vi "RCL.vi"(8 "error in (no error)":errorcluster, 10 "Memory":T1, 11 "refnum in":T2) -> (3 "refnum out":T2, 4 "question out":string)   [LabVIEW 2021, in "Korad KA3305P.lvlib"]
uses:
  Korad KA3305P.lvlib
  Reference.ctl
  MemoryNo.ctl
panel:
  out "error out":errorcluster
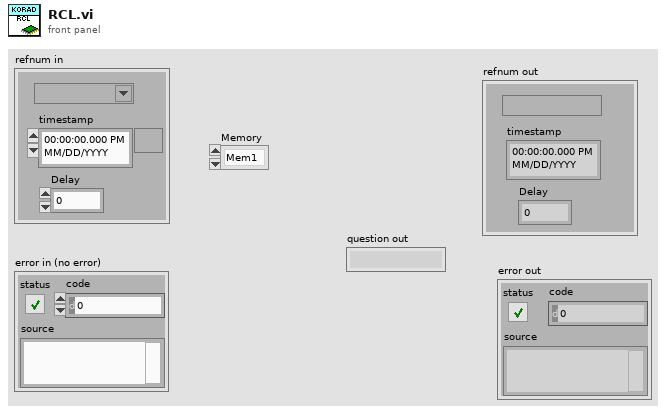
[diagram p1: front panel]
types:
  T1 = typedef "Korad KA3305P.lvlib/MemoryNo.ctl" = enum16{"Mem1", "Mem2", "Mem3", "Mem4", "Mem5"}
  T2 = typedef "Korad KA3305P.lvlib/Reference.ctl" = cluster{"refnum":refnum<visa-resource-name>, "timestamp":timestamp, "Delay":dbl}
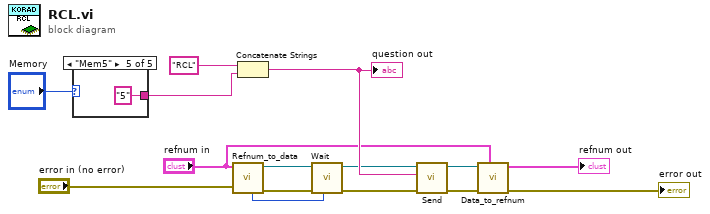
[diagram p0: block diagram]
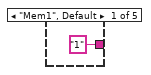
[diagram p2: hidden frame]
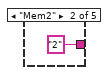
[diagram p3: hidden frame]
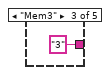
[diagram p4: hidden frame]
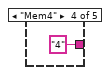
[diagram p5: hidden frame]
diagram:
  n1 = case shown="\"Mem5\"" "Memory" {
    tunnel: ["1" ("string") "2" ("string") "3" ("string") "4" ("string") "5" ("string")] -> w1
    frame "Mem1", Default {
    }
    frame "Mem2" {
    }
    frame "Mem3" {
    }
    frame "Mem4" {
    }
    frame "Mem5" {
    }
  }
  n2 = call "Refnum_to_data.vi"("error in (no error)"="error in (no error)", "refnum in"="refnum in") -> ("error out"=w9:errorcluster, "DAQ refnum out"=w8:refnum<visa-resource-name>, "delay out"=w7:u32)  [unwired: 7 in]
  n3 = Concatenate Strings("RCL" ("string"), w1) -> (w14:string)
  "question out" <- w14
  n4 = call "Wait.vi"("milliseconds to wait"=w7, "error in (no error)"=w9, "refnum in"=w8) -> ("error out"=w13:errorcluster, "refnum out"=w11:refnum<visa-resource-name>)  [unwired: 7 in]
  n5 = call "Send.vi"("error in (no error)"=w13, "data"=w14, "refnum in"=w11) -> ("error out"=w10:errorcluster, "refnum out"=w5:refnum<visa-resource-name>)  [unwired: 7 in]
  n6 = call "Data_to_refnum.vi"("refnum in"="refnum in", "error in (no error)"=w10, "DAQ refnum in"=w5) -> ("error out"=→"error out":errorcluster, "refnum out"=→"refnum out":T2)  [unwired: 7 in]
